vi "Find Bit Depth (SubVI).vi"(0 "Maximum":u8, 2 "Minimum (In)":u8, 5 "Input Valid?":bool) -> (14 "Minimum (Out)":u8, 16 "Bit Depth":u8, 19 "Output Valid?":bool)   [LabVIEW 2015]
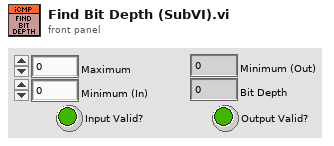
[diagram p1: front panel]
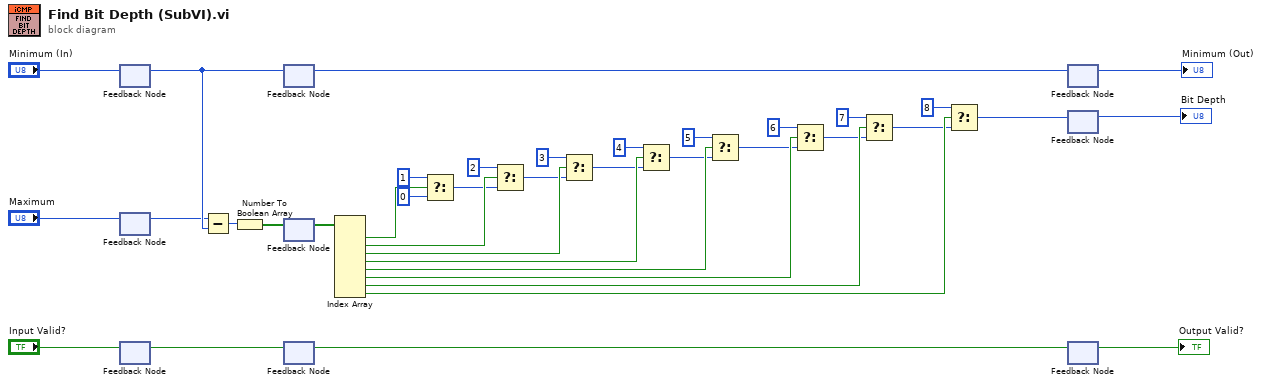
[diagram p0: block diagram]
diagram:
  n1 = feedback-in #1("Minimum (In)") -> ()
  n2 = feedback #1() -> (w6:u8)  [unwired: 1 in]
  n3 = feedback-in #2("Maximum") -> ()
  n4 = feedback #2() -> (w5:u8)  [unwired: 1 in]
  n5 = feedback-in #3("Input Valid?") -> ()
  n6 = feedback #3() -> (w4:bool)  [unwired: 1 in]
  n7 = Subtract(x=w5, y=w6) -> (x-y=w11:u8)
  n8 = Number To Boolean Array(number=w11) -> (Boolean array=w12:bool[])
  n9 = feedback-in #4(w6) -> ()
  n10 = feedback #4() -> (w9:u8)  [unwired: 1 in]
  n11 = feedback-in #5(w12) -> ()
  n12 = feedback #5() -> (w8:bool[])  [unwired: 1 in]
  n13 = feedback-in #6(w4) -> ()
  n14 = feedback #6() -> (w7:bool)  [unwired: 1 in]
  n15 = Index Array(array=w8) -> (element #1=w13:bool, element #2=w17:bool, element #3=w21:bool, element #4=w32:bool, element #5=w33:bool, element #6=w34:bool, element #7=w35:bool, element #8=w36:bool)  [unwired: 8 in]
  n16 = Select(t=u8 1, s=w13, f=u8 0) -> (s? t:f=w16:u8)
  n17 = Select(t=u8 2, s=w17, f=w16) -> (s? t:f=w20:u8)
  n18 = Select(t=u8 3, s=w21, f=w20) -> (s? t:f=w25:u8)
  n19 = Select(t=u8 4, s=w32, f=w25) -> (s? t:f=w22:u8)
  n20 = Select(t=u8 5, s=w33, f=w22) -> (s? t:f=w29:u8)
  n21 = Select(t=u8 6, s=w34, f=w29) -> (s? t:f=w28:u8)
  n22 = Select(t=u8 7, s=w35, f=w28) -> (s? t:f=w31:u8)
  n23 = Select(t=u8 8, s=w36, f=w31) -> (s? t:f=w37:u8)
  n24 = feedback-in #7(w9) -> ()
  n25 = feedback #7() -> (→"Minimum (Out)":u8)  [unwired: 1 in]
  n26 = feedback-in #8(w37) -> ()
  n27 = feedback #8() -> (→"Bit Depth":u8)  [unwired: 1 in]
  n28 = feedback-in #9(w7) -> ()
  n29 = feedback #9() -> (→"Output Valid?":bool)  [unwired: 1 in]
